vi "Get User Attribute.vi"(0 "User Manager Model in":refnum<class "User Manager Model.lvclass">, 5 "Attribute Information":T1, 11 "error in (no error)":errorcluster) -> (4 "User Manager Model out":refnum<class "User Manager Model.lvclass">, 15 "error out":errorcluster)   [LabVIEW 2017, in "User Manager Model.lvlib" / "User Manager Model.lvclass"]
uses:
  User Manager Model.lvclass
  C:/Program Files/National Instruments/LabVIEW 2017/vi.lib/gpm_packages/@cs/mva-core/Source/IModel/IModel/IModel.lvclass
  User Manager Model.lvclass/User Manager Model.ctl
  <vilib>/gpm_packages/@cs/mva-core/Source/IObserver/IObserver/IObserver.lvclass/IObserver.ctl
  <vilib>/gpm_packages/@cs/mva-core/Source/IModel/IModel/IModel.lvclass/IModel.ctl
  <vilib>/gpm_packages/@cs/mva-core/Source/IMediator/PublishRequest/PublishRequest.lvclass/PublishRequest.ctl
  <vilib>/gpm_packages/@cs/mva-core/Source/IMediator/IMediator Messages/Publish Msg/Publish Msg.lvclass/Publish Msg.ctl
  <vilib>/gpm_packages/@cs/actor-framework-messages/Source/RoundTripMessage/RoundTripMessage.lvclass/RoundTripMessage.ctl
  <vilib>/ActorFramework/Message Enqueuer/Message Enqueuer.lvclass/Message Enqueuer.ctl
  <vilib>/gpm_packages/@cs/mva-core/Source/IMediator/IMediator Messages/Publish Msg/Send Pre-Addressed Publish.vi
  <vilib>/gpm_packages/@cs/mva-core/Source/IObserver/IObserver/Read Unique ID.vi
  <vilib>/gpm_packages/@cs/mva-core/Source/IMediator/PublishRequest/Pack Publish Request.vi
  <vilib>/gpm_packages/@cs/actor-framework-messages/Source/RoundTripMessage/Return Round-Trip Message.vi
  <vilib>/ActorFramework/Message Enqueuer/Enqueue.vi
  <vilib>/gpm_packages/@cs/mva-core/Source/IModel/IModel/IModel.lvclass
  C:/Program Files/National Instruments/LabVIEW 2017/vi.lib/gpm_packages/@cs/mva-core/Source/IObserver/IObserver/IObserver.lvclass
  <vilib>/gpm_packages/@cs/mva-core/Source/IMediator/IMediator Messages/Publish Msg/Publish Msg.lvclass
  C:/Program Files/National Instruments/LabVIEW 2017/vi.lib/gpm_packages/@cs/actor-framework-messages/Source/RoundTripMessage/RoundTripMessage.lvclass
  <vilib>/gpm_packages/@cs/actor-framework-messages/Source/RoundTripMessage/RoundTripMessage.lvclass
  C:/Program Files/National Instruments/LabVIEW 2017/vi.lib/ActorFramework/Message/Message.lvclass
  <vilib>/Utility/error.llb/Error Cluster From Error Code.vi
  <vilib>/ActorFramework/Message Priority Queue/Priority Enqueue.vi
  <vilib>/gpm_packages/@cs/mva-core/Source/IMediator/PublishRequest/PublishRequest.lvclass
  <vilib>/gpm_packages/@cs/user-manager/Source/User Configuration Manager Ref/By Ref.lvlib
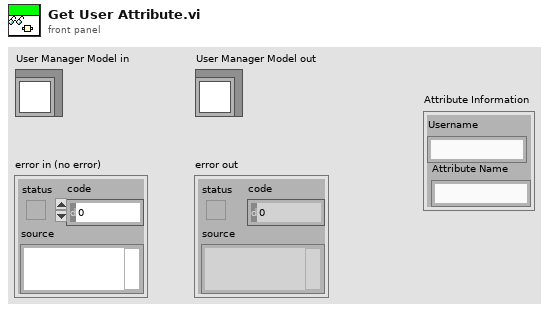
[diagram p1: front panel]
types:
  T1 = cluster{"Username":string, "Attribute Name":string}
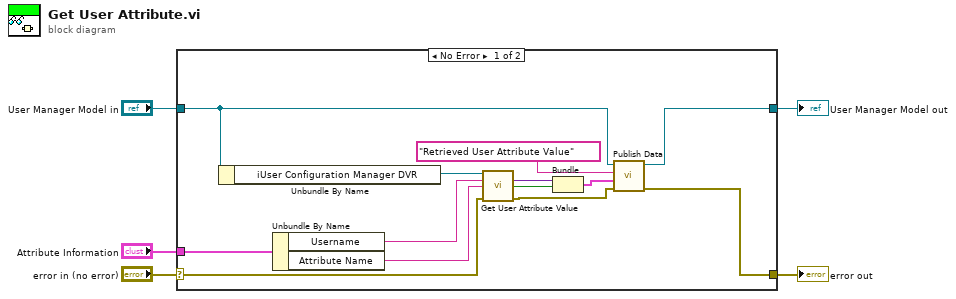
[diagram p0: block diagram]
diagram:
  n1 = case shown="No Error" "error in (no error)" {
    selector: "error in (no error)" -> [w14 w20]
    tunnel: [w6 w20] -> w4
    tunnel: [w8 w19] -> w2
    tunnel: "User Manager Model in" -> [w9 w19]
    tunnel: "Attribute Information" -> [w17 _]
    frame No Error {
      n2 = Unbundle By Name(w9) -> ("iUser Configuration Manager DVR"=w18:refnum<data-value>)
      n3 = Unbundle By Name(w17) -> ("Username"=w16:string, "Attribute Name"=w15:string)
      n4 = call <vilib>:"Get User Attribute Value.vi"("iUser Configuration Manager DVR"=w18, "Username"=w16, "Attribute Name"=w15, "error in"=w14) -> ("Attribute Value"=w13:variant, "Found"=w12:bool, "error out"=w7:errorcluster)  [unwired: 8 in, 1 out]
      n5 = Bundle("Attribute Value"=w13, "Found"=w12) -> (w11:cluster{"Attribute Value":variant, "Found":bool})  [unwired: 1 in]
      n6 = call <vilib>:"Publish Data.vi"("error in (no error)"=w7, "Data to Publish"=w11, "Datum Name"="Retrieved User Attribute Value", "IModel in"=w9) -> ("error out"=w6:errorcluster, "IModel out"=w8:refnum<class "User Manager Model.lvclass">)  [unwired: 6 in]
    }
    frame Error {
    }
  }
  "error out" <- w4
  "User Manager Model out" <- w2
